vi "Get DUT Pins and System Pins from Expanded Pin List.vi"(0 "Expanded Pin Information":T1[](array[typedef])) -> (4 "DUT Pins":T1[](array[typedef]), 6 "System Pins":T1[](array[typedef]))   [LabVIEW 2020]
uses:
  TSM Expanded Pin Information.ctl
  TSM Pin Type Identifier.ctl
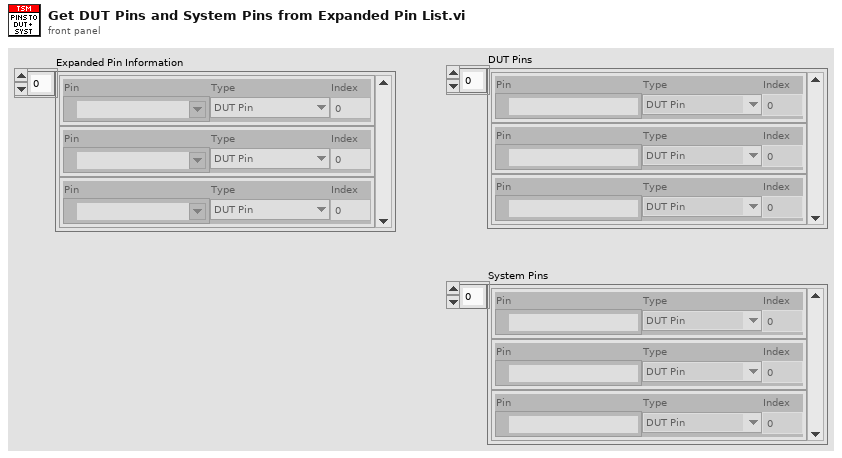
[diagram p1: front panel]
types:
  T1 = typedef "TSM Expanded Pin Information.ctl" = cluster{"Pin":tag, "Type":T2, "Index":i32}
  T2 = typedef "TSM Pin Type Identifier.ctl" = enum8{"DUT Pin", "System Pin", "Pin Group", "Not Determined"}
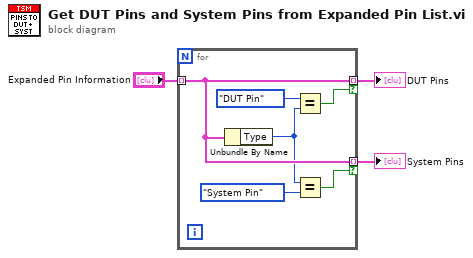
[diagram p0: block diagram]
diagram:
  n1 = for {
    tunnel: "Expanded Pin Information" -> [w9] mode=indexing
    tunnel: [w9] -> w2 mode=indexing if=w4
    tunnel: [w9] -> w1 mode=indexing if=w5
    n2 = Unbundle By Name(w9) -> ("Type"=w8:T2)
    n3 = Equal?(x=TSM_Pin_Type_Identifier."DUT Pin", y=w8) -> (x = y?=w4:bool)
    n4 = Equal?(x=w8, y=TSM_Pin_Type_Identifier."System Pin") -> (x = y?=w5:bool)
  }
  "DUT Pins" <- w2
  "System Pins" <- w1
